vi "Plot Images Property.vi"() -> ()   [LabVIEW 2018]
doc: "This VI demonstrates how to use Plot Images to put a pictures on a Waveform Graph. Plot Images can be positioned behind the grid lines, between the grid lines and plots, or in front of the plots.\n\nThe Plot Images property also works on XY Graphs and Digital Waveform Graphs."
panel:
  in  "Stop":bool
  in  "Back":bool
  in  "Middle":bool
  in  "Front":bool
  out "Waveform Graph":dbl[](graph)
  # "Overview: Demonstrates the use of the Plot Images properties to display custom images at various overlay positions within the plot area of a Waveform Graph, XY Graph, or Digital Waveform Graph.\nInstructions:\n1. Run the VI.\n2. Click the Front, Middle, and Back buttons to show/hide images at different overlay positions.\n3. Click Stop to stop the VI."
  # "Visible Plot Images"
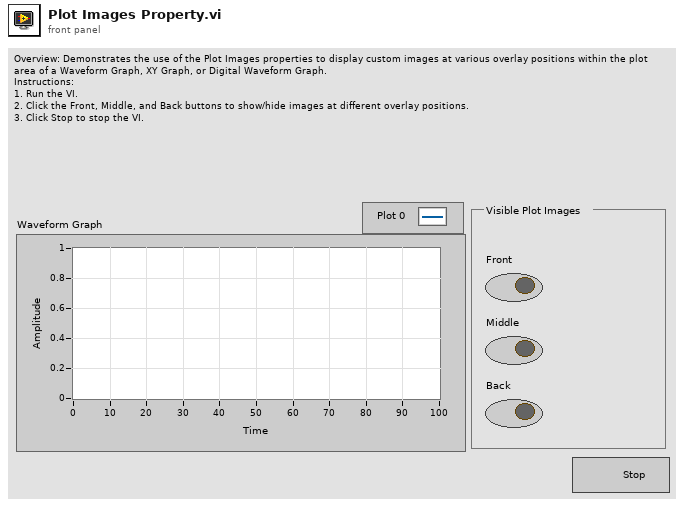
[diagram p1: front panel]
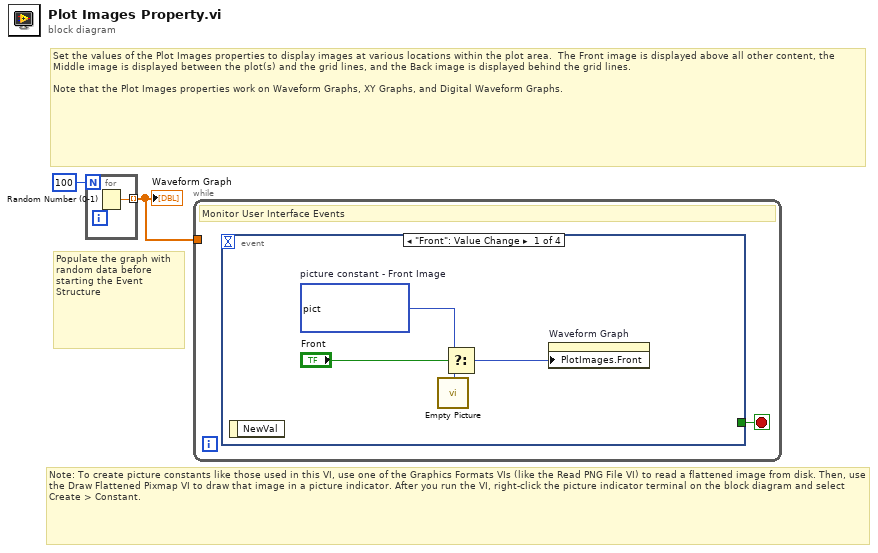
[diagram p0: block diagram]
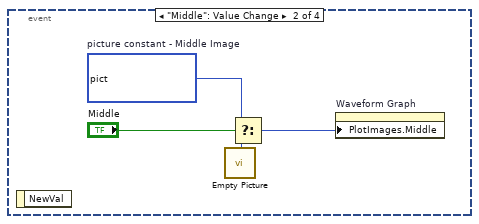
[diagram p2: hidden frame]
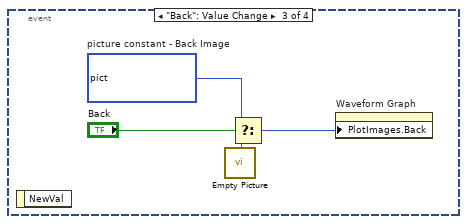
[diagram p3: hidden frame]
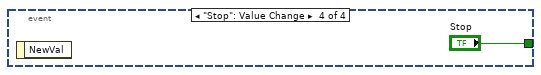
[diagram p4: hidden frame]
diagram:
  # "Note: To create picture constants like those used in this VI, use one of the Graphics Formats VIs (like the Read PNG File VI) to read a flattened image from disk. Then, use the Draw Flattened Pixmap VI to draw that image in a picture indicator. After you run the VI, right-click the picture indicator terminal on the block diagram and select Create > Constant."
  # "Set the values of the Plot Images properties to display images at various locations within the plot area.  The Front image is displayed above all other content, the Middle image is displayed between the plot(s) and the grid lines, and the Back image is displayed behind the grid lines.\n\nNote that the Plot Images properties work on Waveform Graphs, XY Graphs, and Digital Waveform Graphs."
  # "Populate the graph with random data before starting the Event Structure"
  n1 = for {
    N: 100 -> [_]
    tunnel: [w3] -> w1 mode=indexing
    n2 = Random Number (0-1)() -> (number: 0 to 1=w3:dbl)
  }
  "Waveform Graph" <- w1
  n3 = while {
    tunnel: w1 -> [_]
    stop <- w4 stop-if-true
    # "Monitor User Interface Events"
    n4 = event shown="[0] \"Front\": Value Change" {
      selector: _ -> [_ _ _ _]
      dyn-events: _ -> [_ _ _ _]
      timeout: _ -> [_ _ _ _]
      tunnel: [_ _ _ "Stop"] -> w4
      event "Front": Value Change {
        w6 = picture bytes[53567]  # picture constant - Front Image
        n5 = event-data() -> ()  [unwired: 1 in, 1 out]
        n6 = call "Empty Picture"() -> ("empty picture"=w7:picture)
        n7 = Select(t=w6, s="Front", f=w7) -> (s? t:f=w5:picture)
        n8 = property on="Waveform Graph" class="WaveformGraph (strict)"("PlotImages.Front"=w5) -> ()  [unwired: 2 in, 2 out]
      }
      event "Middle": Value Change {
        w11 = picture bytes[167549]  # picture constant - Middle Image
        n9 = event-data() -> ()  [unwired: 1 in, 1 out]
        n10 = call "Empty Picture"() -> ("empty picture"=w12:picture)
        n11 = Select(t=w11, s="Middle", f=w12) -> (s? t:f=w10:picture)
        n12 = property on="Waveform Graph" class="WaveformGraph (strict)"("PlotImages.Middle"=w10) -> ()  [unwired: 2 in, 2 out]
      }
      event "Back": Value Change {
        w15 = picture bytes[179638]  # picture constant - Back Image
        n13 = event-data() -> ()  [unwired: 1 in, 1 out]
        n14 = call "Empty Picture"() -> ("empty picture"=w16:picture)
        n15 = Select(t=w15, s="Back", f=w16) -> (s? t:f=w14:picture)
        n16 = property on="Waveform Graph" class="WaveformGraph (strict)"("PlotImages.Back"=w14) -> ()  [unwired: 2 in, 2 out]
      }
      event "Stop": Value Change {
        n17 = event-data() -> ()  [unwired: 1 in, 1 out]
      }
    }
  }
